vi "Settings_Save.vi"(8 "error in":errorcluster, 11 "DataCluster":T1) -> (0 "error out":errorcluster)   [LabVIEW 2022 SP3]
uses:
  DataCluster.ctl
  <vilib>/Utility/xml.llb/Write to XML File(string).vi
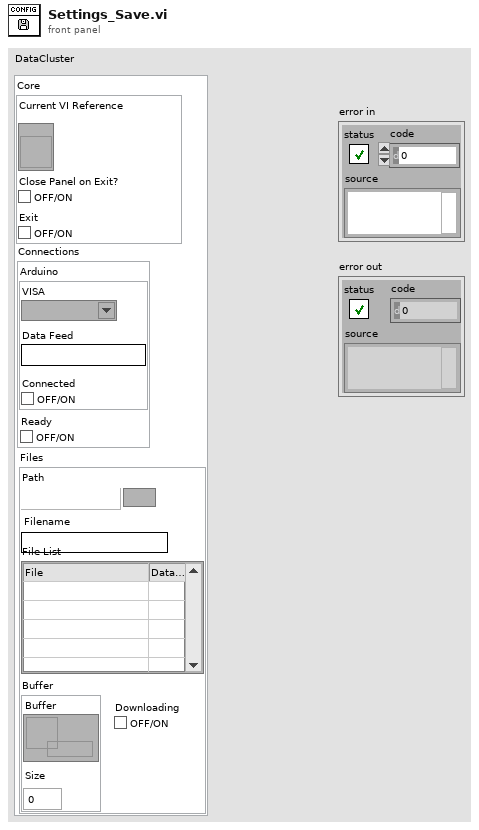
[diagram p1: front panel]
types:
  T1 = typedef "DataCluster.ctl" = cluster{"Core":cluster{"Current VI Reference":refnum<vi>, "Close Panel on Exit?":bool, "Exit":bool}, "Connections":cluster{"Arduino":cluster{"VISA":refnum<visa-resource-name>, "Data Feed":string, "Connected":bool}, "Ready":bool}, "Files":cluster{"Path":path, "Filename":string, "File List":i32, "Buffer":cluster{"Buffer":refnum<queue>, "Size":i32}, "Downloading":bool}}
  T2 = enum16{"open", "replace", "create", "open or create", "replace or create", "replace or create with confirmation"}
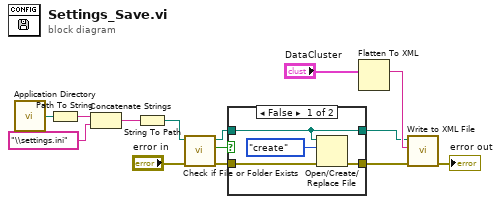
[diagram p0: block diagram]
diagram:
  n1 = call <vilib>:"Application Directory.vi"() -> ("Application Directory"=w12:path)
  n2 = Path To String(path=w12) -> (string=w13:string)
  n3 = Concatenate Strings(w13, "\\settings.ini" ("string")) -> (w10:string)
  n4 = String To Path(string=w10) -> (path=w7:path)
  n5 = call <vilib>:"Check if File or Folder Exists.vi"("error in (no error)"="error in", "path"=w7) -> ("error out"=w3:errorcluster, "file or folder exists?"=w5:bool, "dup path"=w4:path)  [unwired: 7 in]
  n6 = case shown="False" w5 {
    tunnel: w4 -> [w15 w19]
    tunnel: w3 -> [w17 w20]
    tunnel: [w16 w20] -> w2
    tunnel: [w15 w19] -> w1
    frame False {
      n7 = Open/Create/Replace File(file path (use dialog)=w15, error in=w17, operation (0:open)=T2."create") -> (error out=w16:errorcluster)  [unwired: 3 in, 2 out]
    }
    frame True {
    }
  }
  n8 = Flatten To XML(6:"DataCluster") -> (2:w14:string)
  n9 = call-poly <vilib>:"Write to XML File.vi"("error in (no error)"=w2, "XML Input"=w14, "XML File Path"=w1) -> ("error out"=→"error out":errorcluster)  [unwired: 6 in, 2 out]
